vi "適應性控制_輸入權重係數+數位積分_隔振(實際控制).vi"() -> ()   [LabVIEW 2010]
panel:
  in  "Kp":dbl
  in  "I增益":dbl
  out "當下誤差":dbl=0.1 format="%#_13g"
  out "模擬輸入x(t)":dbl[][](graph)
  out "理想與FIR輸出":dbl[][](graph)
  out "message":string=" INSTRUCTIONS:\r\rNormal Use:  When using subVIs that incorporate the error in/error out (or error I/O) structure, place this handler where you want to inform the user of an error, typically at the end of the I/O data path, as the last action of the program.  If the error in error? is ERROR, the handler creates a message describing the error and its source.  If the type of dialog = 1 (default), the message is displayed to the user, who can only acknowedge it.  If the type = 2, the user can acknowledge the message or abort execution; aborting a program with active I/O is not recommended.  If the type = 0, no message is displayed; this is used to process the error programmatically, and the error out cluster elements are wired to individual terminals for that reason.  \r\rOther Use:\n\r\nlocal testing.  To test the error code of a subVI or function that does not have the error I/O structure, you can wire its error code and a source string to the local error code and error source inputs.  If error in error? indicates no error and error code is not equal to 0, the local code and source are substituted for the error in values, and error? is set TRUE (ERROR)."
  out "誤差":dbl(graph)
  out "while平均運行時間":dbl
  out "收斂time":dbl
  out "各頻率誤差已達標準":bool
  in  "各頻率誤差低於多少亮燈":dbl=0.1 format="%#_13g"
  in  "order":i32=100
  in  "取樣頻率":dbl=100.0 min=1.0 max=1000.0 step=1.0
  in  "stop":bool
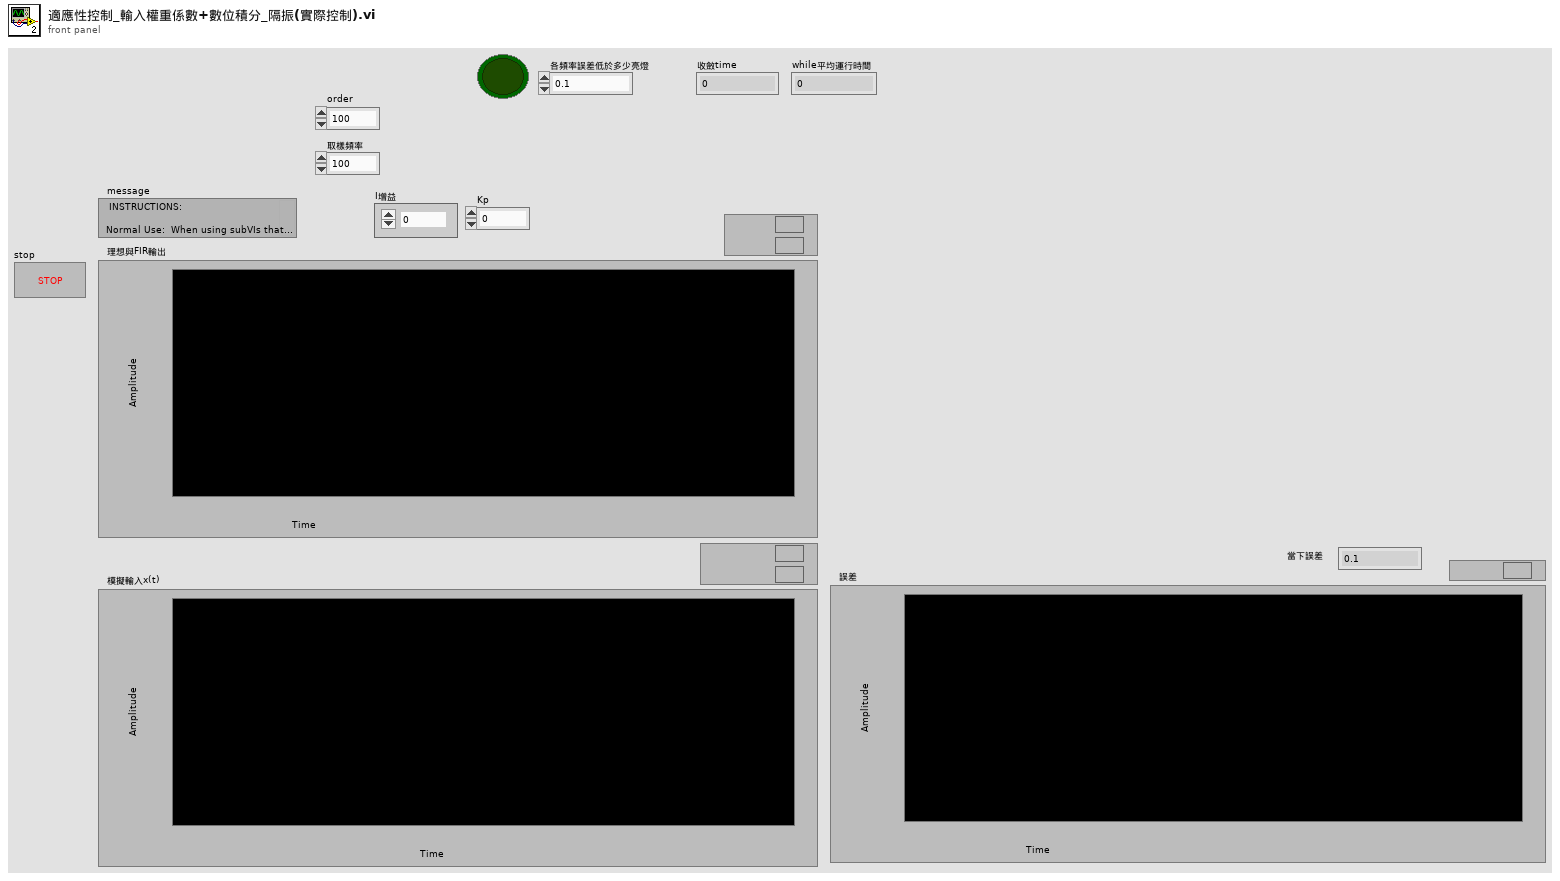
[diagram p1: front panel]
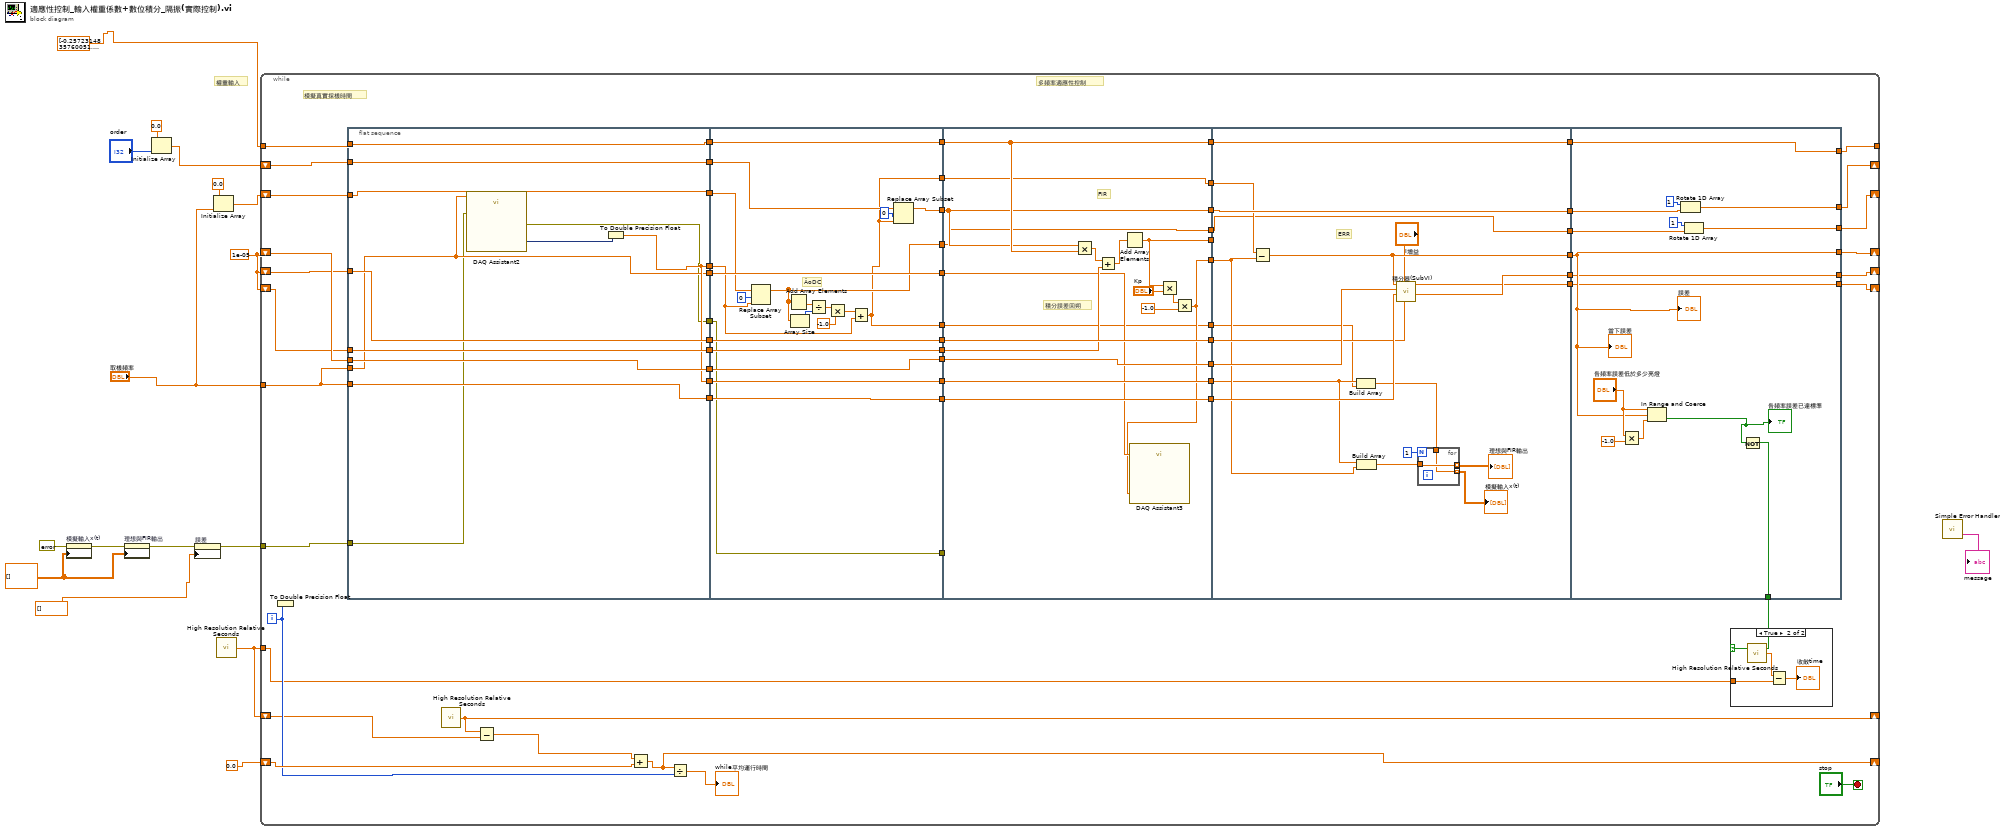
[diagram p0: block diagram]
diagram:
  w7 = 1e-05 ("x")
  w2 = dbl[][] [] ("History Data")
  # "權重輸入"
  n1 = property on="模擬輸入x(t)" class="WFChart (strict)"(error in=errorcluster {"status"=FALSE, "code"=0, "source"=""} ("error constant"), "History Data"=w2) -> (error out=w11:errorcluster)  [unwired: 1 in, 1 out]
  n2 = property on="理想與FIR輸出" class="WFChart (strict)"(error in=w11, "History Data"=w2) -> (error out=w12:errorcluster)  [unwired: 1 in, 1 out]
  n3 = Initialize Array(0.0 ("element"), "order") -> (w6:dbl[])
  n4 = property on="誤差" class="WFChart (strict)"(error in=w12, "History Data"=dbl[] []) -> (error out=w14:errorcluster)  [unwired: 1 in, 1 out]
  n5 = Initialize Array(0.0 ("element"), "取樣頻率") -> (w4:dbl[])
  n6 = call <vilib>:"High Resolution Relative Seconds.vi"() -> ("relative seconds"=w16:dbl)
  n7 = while {
    shift-right: [w54] -> _
    shift-left: w6 -> [w79]
    tunnel: w16 -> [w62]
    shift-right: [w63] -> _
    shift-left: w16 -> [w61]
    shift-right: [w64] -> _
    shift-left: 0.0 -> [w66]
    tunnel: w14 -> [w58]
    shift-right: [w52] -> _
    shift-left: w7 -> [w48]
    shift-right: [w44] -> _
    shift-left: w7 -> [w39]
    shift-right: [w38] -> _
    shift-left: w7 -> [w34]
    tunnel: "取樣頻率" -> [w33]
    tunnel: dbl[] [-0.2572314835760051, -0.2672958503261835, -0.27329046303484417, -0.27512373003724094, -0.27277744646720054, -0.26629549483012704, -0.25578223839396286, -0.2414041777197835, -0.22338352162055186, -0.2019991738147246, -0.1775811082602622, -0.1505042809096985, -0.12118330594564061, -0.09006641393606628, -0.05762754172535077, -0.02436051088728418, 0.00922913159010105, 0.042630865965993095, 0.07533612769399231, 0.1068522609238103] ("權重(w)") -> [w74]
    tunnel: [w26] -> _
    shift-right: [w23] -> _
    shift-left: w4 -> [w25]
    i -> [w65]
    stop <- "stop" stop-if-true
    # "模擬真實採樣時間"
    # "多頻率適應性控制"
    n8 = To Double Precision Float(number=w65) -> ()  [unwired: 1 out]
    n9 = flat-sequence {
      tunnel: [w96] -> w80
      tunnel: w79 -> [w96]
      tunnel: [w89] -> w78
      tunnel: [w95] -> w75
      tunnel: w74 -> [w95]
      tunnel: w58 -> [w86]
      tunnel: [w89] -> w55
      tunnel: [w94] -> w49
      tunnel: w48 -> [w94]
      tunnel: [w93] -> w45
      tunnel: w33 -> [w93]
      tunnel: [w92] -> w40
      tunnel: w39 -> [w92]
      tunnel: [w91] -> w35
      tunnel: w34 -> [w91]
      tunnel: w33 -> [w88]
      tunnel: [w88] -> w32
      tunnel: [w87] -> w31
      tunnel: w25 -> [w85]
      tunnel: [w85] -> w24
      tunnel: w80 -> [w116]
      tunnel: w78 -> [w98]
      tunnel: [w108] -> w77
      tunnel: [w117] -> w76
      tunnel: w75 -> [w117]
      tunnel: [w109] -> w59
      tunnel: [w115] -> w56
      tunnel: w55 -> [w115]
      tunnel: [w113] -> w50
      tunnel: w49 -> [w113]
      tunnel: [w112] -> w46
      tunnel: w45 -> [w112]
      tunnel: [w111] -> w41
      tunnel: w40 -> [w111]
      tunnel: [w110] -> w36
      tunnel: w35 -> [w110]
      tunnel: w32 -> [w107]
      tunnel: w31 -> [w109]
      tunnel: [w107] -> w30
      tunnel: [w97] -> w28
      tunnel: w24 -> [w105]
      tunnel: [w103] -> w20
      tunnel: [w97] -> w19
      tunnel: w77 -> [w133]
      tunnel: w76 -> [w135]
      tunnel: [w135] -> w73
      tunnel: [w126] -> w72
      tunnel: [w133] -> w71
      tunnel: w59 -> [_]
      tunnel: [w134] -> w57
      tunnel: w56 -> [w134]
      tunnel: [w132] -> w51
      tunnel: w50 -> [w132]
      tunnel: [w131] -> w47
      tunnel: w46 -> [w131]
      tunnel: [w130] -> w42
      tunnel: w41 -> [w130]
      tunnel: w36 -> [w128]
      tunnel: w30 -> [w123]
      tunnel: [w122] -> w29
      tunnel: w28 -> [w122]
      tunnel: [w121] -> w27
      tunnel: [w119] -> w21
      tunnel: w20 -> [w119]
      tunnel: w19 -> [w120]
      tunnel: [w120] -> w18
      tunnel: w73 -> [w149]
      tunnel: w72 -> [_]
      tunnel: w71 -> [w151]
      tunnel: [w151] -> w70
      tunnel: [w147] -> w69
      tunnel: w57 -> [w138]
      tunnel: [w149] -> w53
      tunnel: w51 -> [w148]
      tunnel: w47 -> [w146]
      tunnel: [w144] -> w43
      tunnel: w42 -> [w143]
      tunnel: [w142] -> w37
      tunnel: w29 -> [w141]
      tunnel: w27 -> [w140]
      tunnel: [w139] -> w22
      tunnel: w21 -> [w139]
      tunnel: w18 -> [w136]
      tunnel: w70 -> [w165]
      tunnel: [w171] -> w54
      tunnel: w69 -> [w162]
      tunnel: [w167] -> w60
      tunnel: [w163] -> w26
      tunnel: w53 -> [w163]
      tunnel: [w162] -> w52
      tunnel: [w161] -> w44
      tunnel: w43 -> [w161]
      tunnel: [w160] -> w38
      tunnel: w37 -> [w160]
      tunnel: [w158] -> w23
      tunnel: w22 -> [w157]
      frame #0 {
        n10 = call "DAQ Assistant2"("rate"=w88, "error in"=w86) -> ("data"=w90:dynamicdata, "error out"=w87:errorcluster)  [unwired: 14 in, 2 out]
        n11 = To Double Precision Float(number=w90) -> (double precision float=w89:dbl)
      }
      frame #1 {
        # "ÂoDC"
        n12 = Replace Array Subset(array=w105, new element=w98, index=0) -> (w103:dbl[])
        n13 = Add Array Elements(numeric array=w103) -> (sum=w104:dbl)
        n14 = Array Size(array=w103) -> (size(s)=w102:i32)
        n15 = Divide(x=w104, y=w102) -> (x/y=w101:dbl)
        n16 = Multiply(x=w101, y=-1.0) -> (x*y=w99:dbl)
        n17 = Add(x=w99, y=w98) -> (x+y=w97:dbl)
        n18 = Replace Array Subset(array=w116, new element=w97, index=0) -> (w108:dbl[])
      }
      frame #2 {
        # "積分誤差回朔"
        # "FIR"
        n19 = Multiply(x=w133, y=w135) -> (x*y=w129:dbl[])
        n20 = Add(x=w129, y=w128) -> (x+y=w127:dbl[])
        n21 = Add Array Elements(numeric array=w127) -> (sum=w126:dbl)
        n22 = Multiply(x=w126, y="Kp") -> (x*y=w124:dbl)
        n23 = Multiply(x=w124, y=-1.0) -> (x*y=w121:dbl)
        n24 = call "DAQ Assistant3"("data"=w121, "rate"=w123) -> ()  [unwired: 15 in, 3 out]
      }
      frame #3 {
        # "ERR"
        n25 = Subtract(x=w141, y=w140) -> (x-y=w147:dbl)
        n26 = Build Array(w138, w136) -> (w137:dbl[])
        n27 = Build Array(w138, w140) -> (w153:dbl[])
        n28 = call "積分器(SubVI).vi"("輸入累加ERR回朔"=w143, "I增益"="I增益", "samples (Hz)"=w146, "前一個ERR"=w148, "當下ERR"=w147) -> ("輸出累加ERR回朔"=w144:dbl, "積分修正量"=w142:dbl)  [unwired: 5 in]
        n29 = for {
          N: 1 -> [_]
          tunnel: [w156] -> w150 mode=indexing
          tunnel: w153 -> [w156]
          tunnel: [w155] -> w152 mode=indexing
          tunnel: w137 -> [w155]
        }
        "理想與FIR輸出" <- w150
        "模擬輸入x(t)" <- w152
      }
      frame #4 {
        n30 = Multiply(x="各頻率誤差低於多少亮燈", y=-1.0) -> (x*y=w168:dbl)
        n31 = In Range and Coerce(upper limit="各頻率誤差低於多少亮燈", x=w162, lower limit=w168) -> (In Range?=w164:bool)  [unwired: 1 out]
        "各頻率誤差已達標準" <- w164
        n32 = Rotate 1D Array(1:w165, 2:1 ("n")) -> (0:w171:dbl[])
        n33 = Rotate 1D Array(1:w157, 2:1 ("n")) -> (0:w158:dbl[])
        n34 = Not(x=w164) -> (.not. x?=w167:bool)
        "誤差" <- w162
        "當下誤差" <- w162
      }
    }
    n35 = call <vilib>:"High Resolution Relative Seconds.vi"() -> ("relative seconds"=w63:dbl)
    n36 = Subtract(x=w63, y=w61) -> (x-y=w68:dbl)
    n37 = Add(x=w68, y=w66) -> (x+y=w64:dbl)
    n38 = Divide(x=w64, y=w65) -> (x/y=→"while平均運行時間":dbl)
    n39 = case shown="True" w60 {
      tunnel: w62 -> [_ w82]
      frame False {
      }
      frame True {
        n40 = call <vilib>:"High Resolution Relative Seconds.vi"() -> ("relative seconds"=w84:dbl)
        n41 = Subtract(x=w84, y=w82) -> (x-y=→"收斂time":dbl)
      }
    }
  }
  n42 = call <vilib>:"Simple Error Handler.vi"() -> ("message"=→"message":string)  [unwired: 5 in, 4 out]
